vi "ValidateSpectrum.vi"(8 "error in":errorcluster, 11 "connection ID in":refnum<k5>) -> (0 "error out":errorcluster, 1 "Error Info":T2, 2 "OK":bool, 3 "connection ID out":refnum<k5>, 4 "Log String":string, 5 "Validated Spectrum Parameters":T1 {"Step Width" format="%#.3g"})   [LabVIEW 2015, in "ProdigyRemoteControl.lvlib"]
uses:
  ProdigyRemoteControl.lvlib
  DEFINITIONS/DEF_RcError.ctl
  DEFINITIONS/DEF_ValSpectrParas.ctl
  DEFINITIONS/DEF_RcCmd.ctl
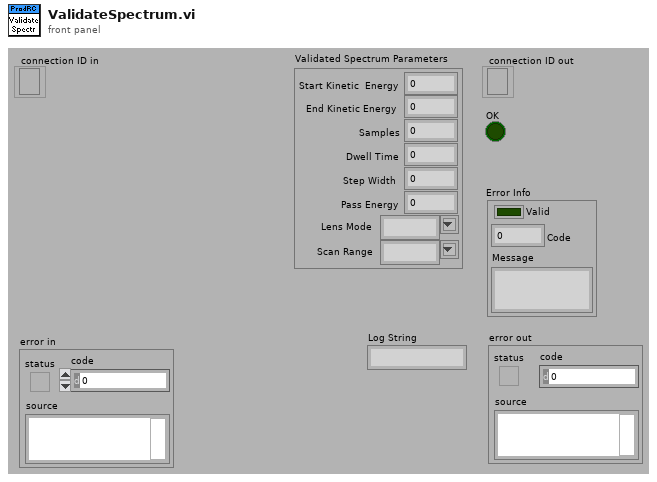
[diagram p1: front panel]
types:
  T1 = typedef "ProdigyRemoteControl.lvlib/DEF_ValSpectrParas.ctl" = cluster{"Start Kinetic  Energy":dbl, "End Kinetic Energy":dbl, "Samples":u32, "Dwell Time":dbl, "Step Width":dbl, "Pass Energy":dbl, "Lens Mode":string, "Scan Range":string}
  T2 = typedef "ProdigyRemoteControl.lvlib/DEF_RcError.ctl" = cluster{"Valid":bool, "Code":u16, "Message":string}
  T3 = typedef "ProdigyRemoteControl.lvlib/DEF_RcCmd.ctl" = string
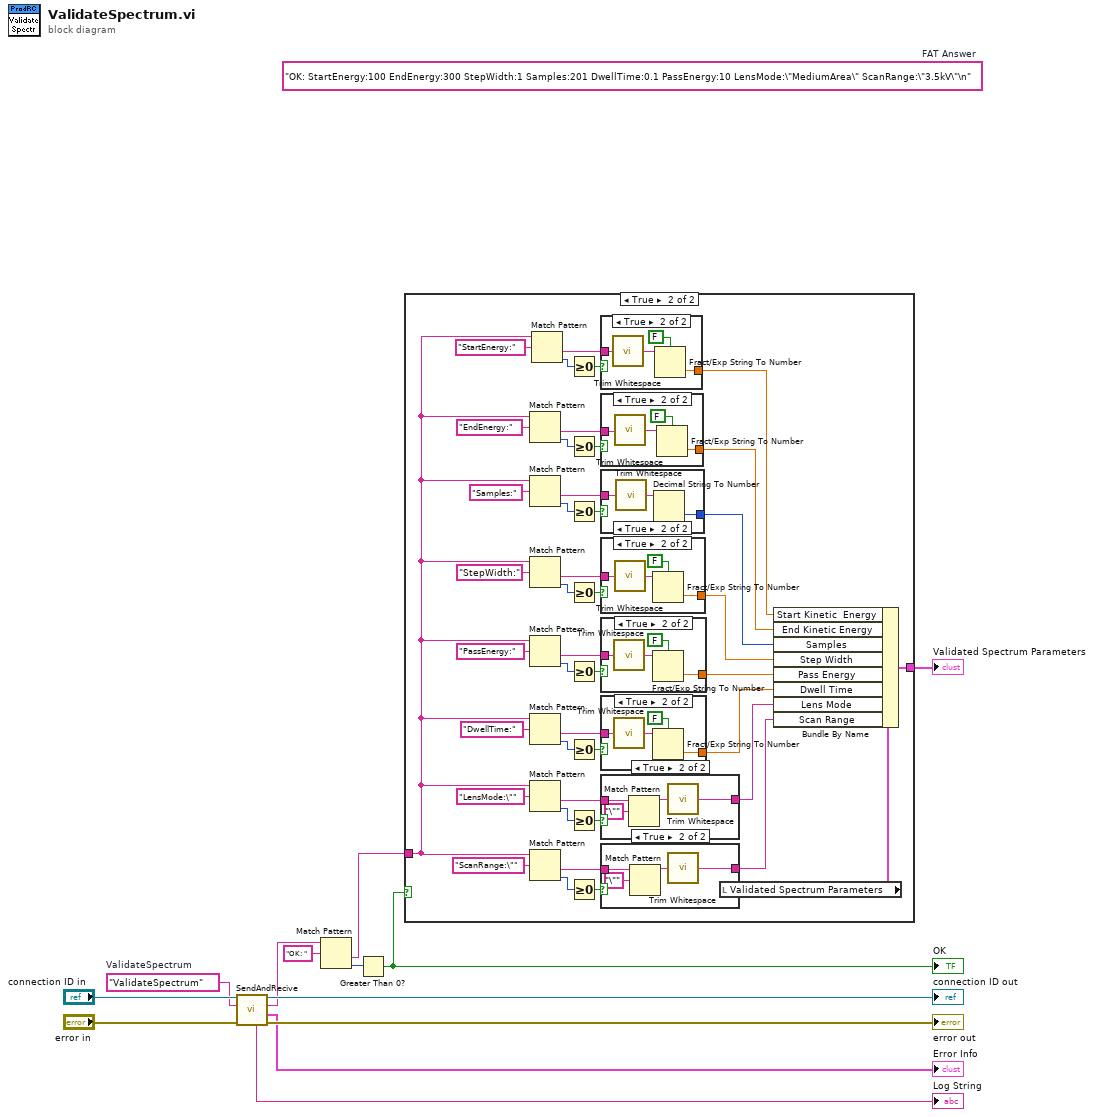
[diagram p0: block diagram]
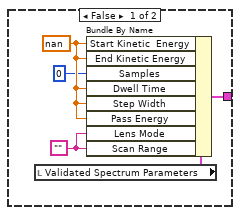
[diagram p2: hidden frame]
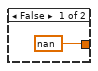
[diagram p3: hidden frame]
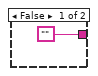
[diagram p4: hidden frame]
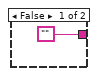
[diagram p5: hidden frame]
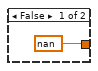
[diagram p6: hidden frame]
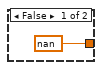
[diagram p7: hidden frame]
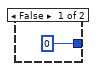
[diagram p8: hidden frame]
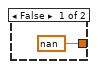
[diagram p9: hidden frame]
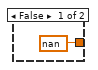
[diagram p10: hidden frame]
diagram:
  (unwired) "OK: StartEnergy:100 EndEnergy:300 StepWidth:1 Samples:201 DwellTime:0.1 PassEnergy:10 LensMode:\"MediumArea\" ScanRange:\"3.5kV\"\n"  # FAT Answer
  w9 = T3 "ValidateSpectrum"  # ValidateSpectrum
  n1 = call "SendAndRecive.vi"("error in"="error in", "Command"=w9, "connection ID in"="connection ID in") -> ("error out"=→"error out":errorcluster, "Error Info"=→"Error Info":T2, "Answer"=w6:string, "connection ID out"=→"connection ID out":refnum<k5>, "Log String"=→"Log String":string)  [unwired: 4 in]
  n2 = Match Pattern(string=w6, regular expression="OK: ") -> (after substring=w2:string, offset past match=w4:i32)  [unwired: 1 in, 2 out]
  n3 = Greater Than 0?(x=w4) -> (x > 0?=w1:bool)
  "OK" <- w1
  n4 = case shown="True" w1 {
    tunnel: w2 -> [_ w19]
    tunnel: [w17 w47] -> w3
    frame False {
      w14 = ""
      w16 = nan ("Start Kinetic  Energy")
      n5 = local read "Validated Spectrum Parameters"() -> (w18:T1)
      n6 = Bundle By Name(cluster=w18, "Start Kinetic  Energy"=w16, "End Kinetic Energy"=w16, "Samples"=u32 0, "Dwell Time"=w16, "Step Width"=w16, "Pass Energy"=w16, "Lens Mode"=w14, "Scan Range"=w14) -> (w17:T1)
    }
    frame True {
      n7 = Match Pattern(string=w19, regular expression="EndEnergy:") -> (after substring=w55:string, offset past match=w54:i32)  [unwired: 1 in, 2 out]
      n8 = Match Pattern(string=w19, regular expression="Samples:") -> (after substring=w52:string, offset past match=w51:i32)  [unwired: 1 in, 2 out]
      n9 = Match Pattern(string=w19, regular expression="StepWidth:") -> (after substring=w49:string, offset past match=w50:i32)  [unwired: 1 in, 2 out]
      n10 = Match Pattern(string=w19, regular expression="PassEnergy:") -> (after substring=w44:string, offset past match=w45:i32)  [unwired: 1 in, 2 out]
      n11 = Match Pattern(string=w19, regular expression="DwellTime:") -> (after substring=w25:string, offset past match=w24:i32)  [unwired: 1 in, 2 out]
      n12 = Match Pattern(string=w19, regular expression="LensMode:\"") -> (after substring=w39:string, offset past match=w38:i32)  [unwired: 1 in, 2 out]
      n13 = Match Pattern(string=w19, regular expression="ScanRange:\"") -> (after substring=w36:string, offset past match=w37:i32)  [unwired: 1 in, 2 out]
      n14 = Match Pattern(string=w19, regular expression="StartEnergy:") -> (after substring=w58:string, offset past match=w60:i32)  [unwired: 1 in, 2 out]
      n15 = Greater Or Equal To 0?(x=w60) -> (x >= 0?=w59:bool)
      n16 = Greater Or Equal To 0?(x=w54) -> (x >= 0?=w57:bool)
      n17 = Greater Or Equal To 0?(x=w51) -> (x >= 0?=w53:bool)
      n18 = Greater Or Equal To 0?(x=w50) -> (x >= 0?=w48:bool)
      n19 = Greater Or Equal To 0?(x=w45) -> (x >= 0?=w42:bool)
      n20 = Greater Or Equal To 0?(x=w24) -> (x >= 0?=w26:bool)
      n21 = Greater Or Equal To 0?(x=w38) -> (x >= 0?=w41:bool)
      n22 = Greater Or Equal To 0?(x=w37) -> (x >= 0?=w34:bool)
      n23 = case shown="True" w59 {
        tunnel: w58 -> [_ w100]
        tunnel: [nan w98] -> w33
        frame False {
        }
        frame True {
          n24 = call <vilib>:"Trim Whitespace.vi"("string"=w100) -> ("trimmed string"=w99:string)  [unwired: 1 in]
          n25 = Fract/Exp String To Number(use system decimal point (T)=FALSE, string=w99) -> (number=w98:dbl)  [unwired: 2 in, 1 out]
        }
      }
      n26 = case shown="True" w57 {
        tunnel: w55 -> [_ w95]
        tunnel: [nan w92] -> w32
        frame False {
        }
        frame True {
          n27 = call <vilib>:"Trim Whitespace.vi"("string"=w95) -> ("trimmed string"=w94:string)  [unwired: 1 in]
          n28 = Fract/Exp String To Number(use system decimal point (T)=FALSE, string=w94) -> (number=w92:dbl)  [unwired: 2 in, 1 out]
        }
      }
      n29 = case shown="True" w53 {
        tunnel: w52 -> [_ w90]
        tunnel: [0 w88] -> w30
        frame False {
        }
        frame True {
          n30 = call <vilib>:"Trim Whitespace.vi"("string"=w90) -> ("trimmed string"=w89:string)  [unwired: 1 in]
          n31 = Decimal String To Number(string=w89) -> (number=w88:i32)  [unwired: 2 in, 1 out]
        }
      }
      n32 = case shown="True" w48 {
        tunnel: w49 -> [_ w86]
        tunnel: [nan w83] -> w28
        frame False {
        }
        frame True {
          n33 = call <vilib>:"Trim Whitespace.vi"("string"=w86) -> ("trimmed string"=w84:string)  [unwired: 1 in]
          n34 = Fract/Exp String To Number(use system decimal point (T)=FALSE, string=w84) -> (number=w83:dbl)  [unwired: 2 in, 1 out]
        }
      }
      n35 = case shown="True" w42 {
        tunnel: w44 -> [_ w81]
        tunnel: [nan w78] -> w27
        frame False {
        }
        frame True {
          n36 = call <vilib>:"Trim Whitespace.vi"("string"=w81) -> ("trimmed string"=w79:string)  [unwired: 1 in]
          n37 = Fract/Exp String To Number(use system decimal point (T)=FALSE, string=w79) -> (number=w78:dbl)  [unwired: 2 in, 1 out]
        }
      }
      n38 = case shown="True" w26 {
        tunnel: w25 -> [_ w66]
        tunnel: [nan w63] -> w22
        frame False {
        }
        frame True {
          n39 = call <vilib>:"Trim Whitespace.vi"("string"=w66) -> ("trimmed string"=w64:string)  [unwired: 1 in]
          n40 = Fract/Exp String To Number(use system decimal point (T)=FALSE, string=w64) -> (number=w63:dbl)  [unwired: 2 in, 1 out]
        }
      }
      n41 = case shown="True" w41 {
        tunnel: w39 -> [_ w76]
        tunnel: ["" w75] -> w21
        frame False {
        }
        frame True {
          n42 = Match Pattern(string=w76, regular expression="\"") -> (before substring=w74:string)  [unwired: 1 in, 3 out]
          n43 = call <vilib>:"Trim Whitespace.vi"("string"=w74) -> ("trimmed string"=w75:string)  [unwired: 1 in]
        }
      }
      n44 = case shown="True" w34 {
        tunnel: w36 -> [_ w71]
        tunnel: ["" w70] -> w20
        frame False {
        }
        frame True {
          n45 = Match Pattern(string=w71, regular expression="\"") -> (before substring=w69:string)  [unwired: 1 in, 3 out]
          n46 = call <vilib>:"Trim Whitespace.vi"("string"=w69) -> ("trimmed string"=w70:string)  [unwired: 1 in]
        }
      }
      n47 = local read "Validated Spectrum Parameters"() -> (w46:T1)
      n48 = Bundle By Name(cluster=w46, "Start Kinetic  Energy"=w33, "End Kinetic Energy"=w32, "Samples"=w30, "Step Width"=w28, "Pass Energy"=w27, "Dwell Time"=w22, "Lens Mode"=w21, "Scan Range"=w20) -> (w47:T1)
    }
  }
  "Validated Spectrum Parameters" <- w3
